vi "resistanceScan.vi"(8 "error in (no error)":errorcluster, 10 "Imax":string, 11 "VISA Refnum in":refnum<visa-resource-name>) -> (0 "error out":errorcluster, 1 "RESISTANCE/CURRENT":cluster{dbl, dbl}(graph), 3 "ADC value":dbl, 4 "overCurrent":bool, 5 "Istring#":string)   [LabVIEW 2018]
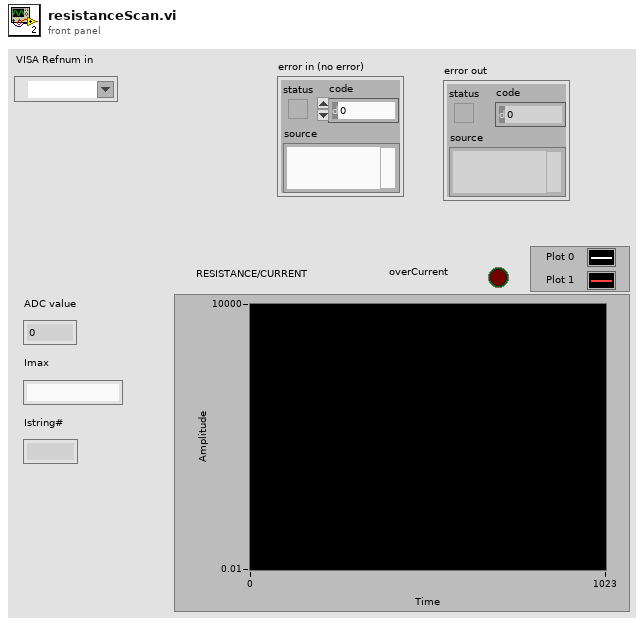
[diagram p1: front panel]
types:
  T1 = cluster{"double precision float":dbl, "Ichart":dbl}
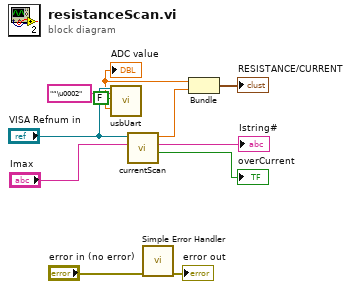
[diagram p0: block diagram]
diagram:
  n1 = call "usbUart.vi"("VISA resource name"="VISA Refnum in", "write buffer"="“\u0002" ("write buffer buffer"), "sdFeature"=FALSE) -> ("double precision float"=w10:dbl)  [unwired: 1 in, 15 out]
  "ADC value" <- w10
  n2 = call "currentScan.vi"("Imax"="Imax", "VISA resource name"="VISA Refnum in") -> ("max"=→"overCurrent":bool, "Istring"=→"Istring#":string, "Ichart"=w2:dbl)  [unwired: 6 in, 1 out]
  n3 = call <vilib>:"Simple Error Handler.vi"("error in (no error)"="error in (no error)") -> ("error out"=→"error out":errorcluster)  [unwired: 4 in, 4 out]
  n4 = Bundle("double precision float"=w10, "Ichart"=w2) -> (→"RESISTANCE/CURRENT":T1)  [unwired: 1 in]
